vi "nonreentrant safe state.vi"(8 "error in (no error)":errorcluster, 9 "result allocation":T1, 10 "parameters":T1, 11 "CVT runtime in":refnum<class "testmod runtime.lvclass">) -> (0 "error out":errorcluster, 1 "results":T1, 2 "parameter allocation":T1)   [LabVIEW 2013, in "testmod runtime.lvclass"]
uses:
  testmod runtime.lvclass
  <vilib>/NI/Tag Bus/table/data table.ctl
  testmod runtime.lvclass/testmod runtime.ctl
  <vilib>/NI/Tag Bus/table/data table.lvlib
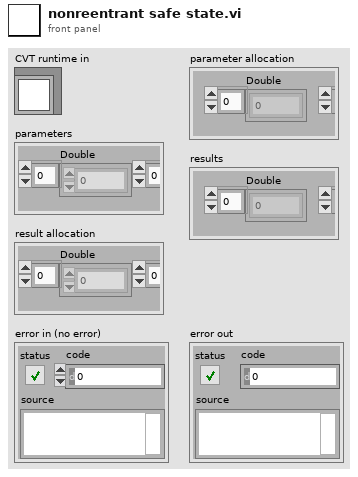
[diagram p1: front panel]
types:
  T1 = typedef "tag bus.lvlib/data table.lvlib/data table.ctl" = cluster{"Double":dbl[], "Single":sgl[], "I64":i64[], "I32":i32[], "I16":i16[], "I8":i8[], "U64":u64[], "U32":u32[], "U16":u16[], "U8":u8[], "Boolean":bool[], "String":string[], "Array of Double":cluster{"DBL Array":dbl[]}[], "Array of Single":cluster{"SGL Array":sgl[]}[], "Array of I64":cluster{"I64 Array":i64[]}[], "Array of I32":cluster{"I32 Array":i32[]}[], "Array of I16":cluster{"I16 Array":i16[]}[], "Array of I8":cluster{"I8 Array":i8[]}[], "Array of U64":cluster{"U64 Array":u64[]}[], "Array of U32":cluster{"U32 Array":u32[]}[], "Array of U16":cluster{"U16 Array":u16[]}[], "Array of U8":cluster{"U8 Array":u8[]}[], "Array of Boolean":cluster{"Boolean Array":bool[]}[], "Array of String":cluster{"String Array":string[]}[]}
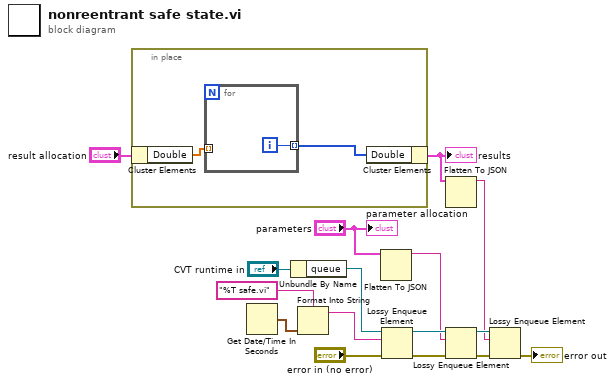
[diagram p0: block diagram]
diagram:
  n1 = in-place {
    n2 = in-place-cluster #1("result allocation") -> ("Double"=w18:dbl[])
    n3 = for {
      tunnel: w18 -> [_] mode=indexing
      tunnel: [w19] -> w17 mode=indexing
      i -> [w19]
    }
    n4 = in-place-cluster #1("Double"=w17) -> (w1:T1)
  }
  "results" <- w1
  n5 = Get Date/Time In Seconds() -> (seconds since 1Jan1904=w11:timestamp)
  n6 = Unbundle By Name("CVT runtime in") -> ("queue"=w14:refnum<queue>)
  n7 = Format Into String(format string="%T safe.vi", w11) -> (resulting string=w10:string)  [unwired: 2 in, 1 out]
  n8 = Flatten To JSON(anything="parameters") -> (JSON string=w3:string)  [unwired: 2 in, 1 out]
  n9 = Lossy Enqueue Element(queue=w14, element=w10, error in (no error)="error in (no error)") -> (queue out=w6:refnum<queue>, error out=w16:errorcluster)  [unwired: 2 out]
  n10 = Flatten To JSON(anything=w1) -> (JSON string=w4:string)  [unwired: 2 in, 1 out]
  n11 = Lossy Enqueue Element(queue=w6, element=w3, error in (no error)=w16) -> (queue out=w5:refnum<queue>, error out=w7:errorcluster)  [unwired: 2 out]
  n12 = Lossy Enqueue Element(queue=w5, element=w4, error in (no error)=w7) -> (error out=→"error out":errorcluster)  [unwired: 3 out]
  "parameter allocation" <- "parameters"
